vi "Set Global LogType Filter.vi"(10 "Group:LogType":T1[](array[typedef]), 11 "GlobalLogFilter in":refnum<class "GlobalLogFilter.lvclass">) -> (3 "GlobalLogFilter out":refnum<class "GlobalLogFilter.lvclass">)   [LabVIEW 2017, in "GlobalLogFilter.lvclass"]
uses:
  GlobalLogFilter.lvclass
  _Support/Typedef/_CSM_GlobalLog_MSG_TYPE.ctl
  GlobalLogFilter.lvclass/GlobalLogFilter.ctl
  Communicable State Machine.lvlib
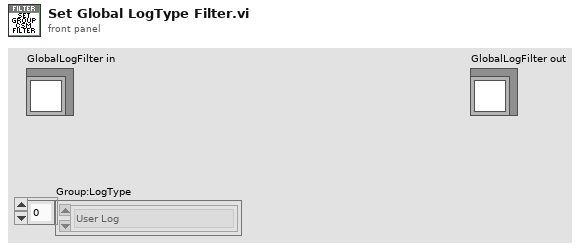
[diagram p1: front panel]
types:
  T1 = typedef "Communicable State Machine.lvlib/_CSM_GlobalLog_MSG_TYPE.ctl" = enum16{"User Log", "State Change", "Status", "Interrupt", "Register", "Unregister", "Error Log", "Module Created", "Module Destroyed"}
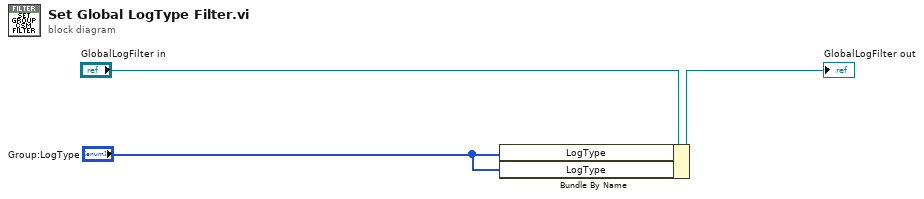
[diagram p0: block diagram]
diagram:
  n1 = Bundle By Name(cluster="GlobalLogFilter in", "LogType"="Group:LogType", "LogType"="Group:LogType") -> (→"GlobalLogFilter out":refnum<class "GlobalLogFilter.lvclass">)
